vi "Cal Freq.vi"(7 "sample":u32, 9 "voltage_resolution":dbl, 10 "buffer_length":u32, 11 "buffer":dbl) -> (2 "function return":dbl, 3 "buffer out":dbl)   [LabVIEW 2021, in "vmmso.lvlib"]
doc: "DLL_API double WINAPI CalFreq(double* buffer, unsigned int buffer_length, double voltage_resolution, unsigned int sample);"
uses:
  vmmso.lvlib
  vmmso.dll
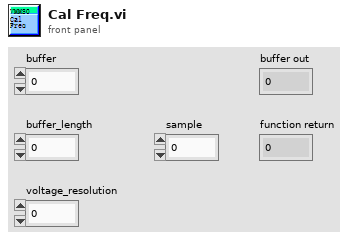
[diagram p1: front panel]
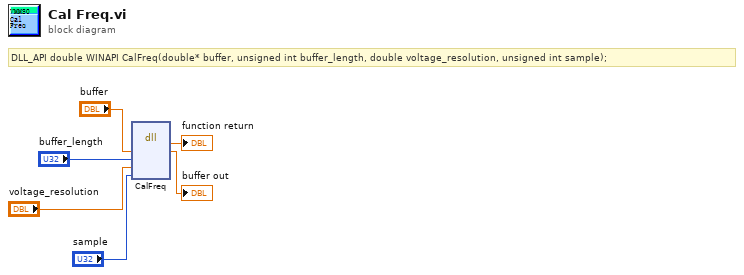
[diagram p0: block diagram]
diagram:
  # "DLL_API double WINAPI CalFreq(double* buffer, unsigned int buffer_length, double voltage_resolution, unsigned int sample);"
  n1 = dll-call lib="D:/labviewdemo/LabviewDemo 21/vmmso/vmmso.*" fn="CalFreq"("buffer"="buffer", "buffer_length"="buffer_length", "voltage_resolution"="voltage_resolution", "sample"="sample") -> (→"function return":dbl, "buffer"=→"buffer out":dbl)  [unwired: 6 in, 2 out]
